vi "状态栏-插入状态信息-35点监测专用.vi"(8 "消息内容":string, 11 "状态类型":enum16{"全部", "报警", "通信", "设置"}(ring)=enum."报警") -> ()   [LabVIEW 2017]
panel:
  out "状态消息":string caption="结果"
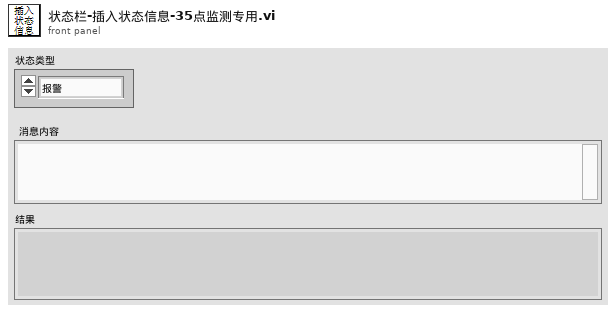
[diagram p1: front panel]
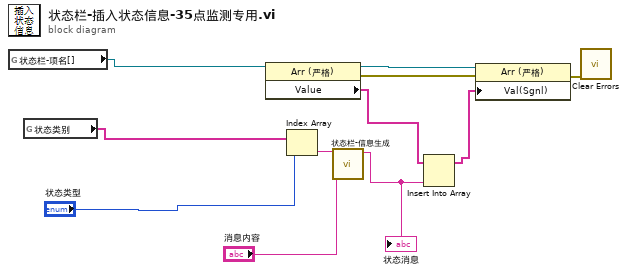
[diagram p0: block diagram]
diagram:
  n1 = global read "全局变量-35点监测.vi" "状态栏-项名[]"() -> (w3:refnum<vi>)
  n2 = global read "全局变量-35点监测.vi" "状态类别"() -> (w2:string[])
  n3 = property on="属性节点" class="Arr (严格)"(reference=w3) -> (reference out=w8:refnum<vi>, error out=w5:errorcluster, "Value"=w7:string[])  [unwired: 1 in]
  n4 = Index Array(array=w2, index="状态类型") -> (element=w10:string)
  n5 = call "状态栏-信息生成.vi"("消息内容"="消息内容", "消息类型"=w10) -> ("状态消息"=w9:string)  [unwired: 9 in]
  "状态消息" <- w9
  n6 = Insert Into Array(array=w7, new element=w9) -> (w11:string[])  [unwired: 1 in]
  n7 = property on="属性节点" class="Arr (严格)"(reference=w8, error in=w5, "Val(Sgnl)"=w11) -> (error out=w4:errorcluster)  [unwired: 1 out]
  n8 = call <vilib>:"Clear Errors.vi"("error in (no error)"=w4) -> ()  [unwired: 5 in, 2 out]
